vi "Publish (async) JSON.vi"(4 "ArgumentsKw":string, 6 "Arguments":string, 7 "Options":string, 8 "Error in":errorcluster, 9 "Notify result":bool, 10 "Topic":string, 11 "WAMP Client in":refnum<class "WAMP Client.lvclass">) -> (0 "Error cout":errorcluster, 2 "notifier out":refnum<notifier>, 3 "WAMP Client out":refnum<class "WAMP Client.lvclass">)   [LabVIEW 2020, in "wamplv.lvlib" / "WAMP Client.lvclass"]
uses:
  WAMP Client.lvclass
  Private/TypeDef/Internal Message Type.ctl
  Private/TypeDef/PUBLISH result (JSON).ctl
  wamplv.lvlib
  Private/TypeDef/PUBLISH Request Data (JSON).ctl
  TypeDefs/Error or abort detail (JSON).ctl
  56cb05c7-ccfa-42e5-a428-2bd237dbc257.vi
  Private/Requests/IInternalMessage/IInternalMessage.lvclass
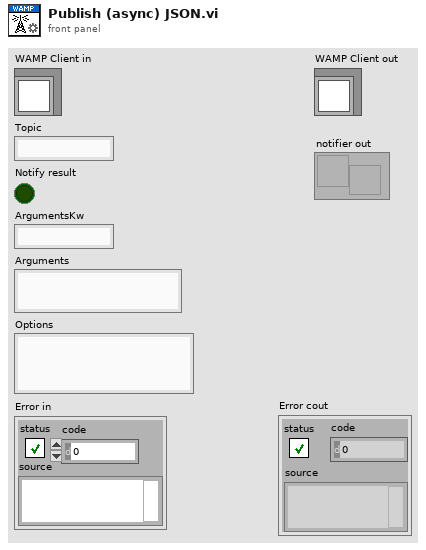
[diagram p1: front panel]
types:
  T1 = typedef "wamplv.lvlib/PUBLISH result (JSON).ctl" = cluster{"Publication ID":u64, "Success?":bool, "Error/Abort details (JSON)":T2}
  T2 = typedef "wamplv.lvlib/Error or abort detail (JSON).ctl" = cluster{"Error URI":string, "Error Arguments":string, "Error ArgumentKw":string, "Error Details":string}
  T3 = typedef "wamplv.lvlib/PUBLISH Request Data (JSON).ctl" = cluster{"Topic URI":string, "Arguments":string, "ArgumentsKw":string, "Request Acknowledgement":bool, "Options":string, "Publish result notifier":refnum<notifier>}
  T4 = typedef "wamplv.lvlib/WAMP Client.lvclass/Internal Message Type.ctl" = enum16{"Subscribe", "Handle Subscribed", "Handle Event", "Unsubscribe", "Handle Unsubscribed", "Publish", "Handled Published", "Goodbye", "Handle Goodbye", "Call", "Handle Result", "Register", "Handle Registered", "Unregister", "Handle Unregistered", "Handle Invocation", "Yield", "Error"}
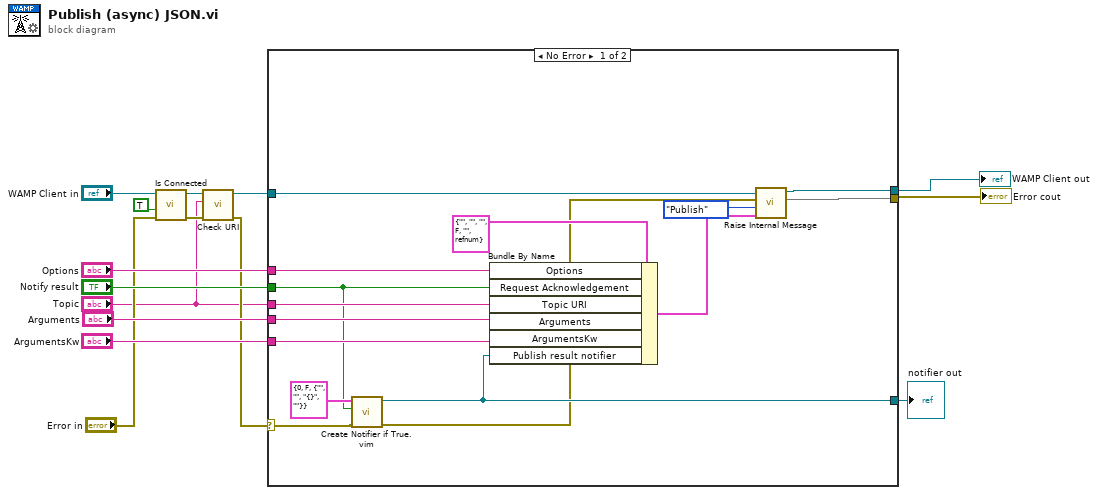
[diagram p0: block diagram]
diagram:
  n1 = call "Is Connected.vi"("error in"="Error in", "Raise error if not connected"=TRUE, "WAMP Client in"="WAMP Client in") -> ("error out"=w5:errorcluster, "WAMP Client out"=w6:refnum<class "WAMP Client.lvclass">)  [unwired: 6 in, 1 out]
  n2 = call "Check URI.vi"("error in (no error)"=w5, "URI"="Topic", "WAMP Client in"=w6) -> ("error out"=w4:errorcluster, "WAMP Client out"=w2:refnum<class "WAMP Client.lvclass">)  [unwired: 5 in, 2 out]
  n3 = case shown="No Error" w4 {
    selector: w4 -> [w18 w32]
    tunnel: [w25 w32] -> w15
    tunnel: [w24 w31] -> w14
    tunnel: w2 -> [w30 w31]
    tunnel: "Topic" -> [w28 _]
    tunnel: "Arguments" -> [w23 _]
    tunnel: "ArgumentsKw" -> [w22 _]
    tunnel: "Notify result" -> [w16 _]
    tunnel: "Options" -> [w21 _]
    tunnel: [w20 _] -> w9
    frame No Error {
      n4 = call "Create Notifier if True.vim"("error in (no error)"=w18, "Boolean"=w16, "RESULT Payload"=T1 {"Publication ID"=0, "Success?"=FALSE, "Error/Abort details (JSON)"={"Error URI"="", "Error Arguments"="", "Error ArgumentKw"="{}", "Error Details"=""}} ("Cluster")) -> ("error out"=w19:errorcluster, "Notifier out"=w20:refnum<notifier>)  [unwired: 7 in]
      n5 = Bundle By Name(cluster=T3 {"Topic URI"="", "Arguments"="", "ArgumentsKw"="", "Request Acknowledgement"=FALSE, "Options"="", "Publish result notifier"=refnum} ("Cluster"), "Options"=w21, "Request Acknowledgement"=w16, "Topic URI"=w28, "Arguments"=w23, "ArgumentsKw"=w22, "Publish result notifier"=w20) -> (w29:T3)
      n6 = call "Raise Internal Message.vi"("error in (no error)"=w29, 9:Internal_Message_Type."Publish" ("Internal Message Type"), "IInternalMessage"=w19, "WAMP Client in"=w30) -> (2:w25, "WAMP Client out"=w24:refnum<class "WAMP Client.lvclass">)  [unwired: 5 in, 1 out]
    }
    frame Error {
    }
  }
  "Error cout" <- w15
  "WAMP Client out" <- w14
  "notifier out" <- w9
